vi "Main Menu - Behavioral Study.vi"() -> ()   [LabVIEW 2012]
uses:
  subVIs/Global_var.vi
  <userlib>/dhd_sdk7/dhd_sdk7.lvlib
panel:
  out "Please wait...":u16(slide) scale=0.0..2000.0
  in  "step4":bool
  in  "Setting":bool
  in  "step3":bool
  in  "step2":bool
  out "error out":errorcluster
  out "stripped path":path
  out "DeviceID":bool
  in  "step1":bool
  in  "stop":bool
  out "Patient's ID":string
  # "Somatosensory Training Protocol\n\n(coded by ananda)  ver1.3, April 2017"
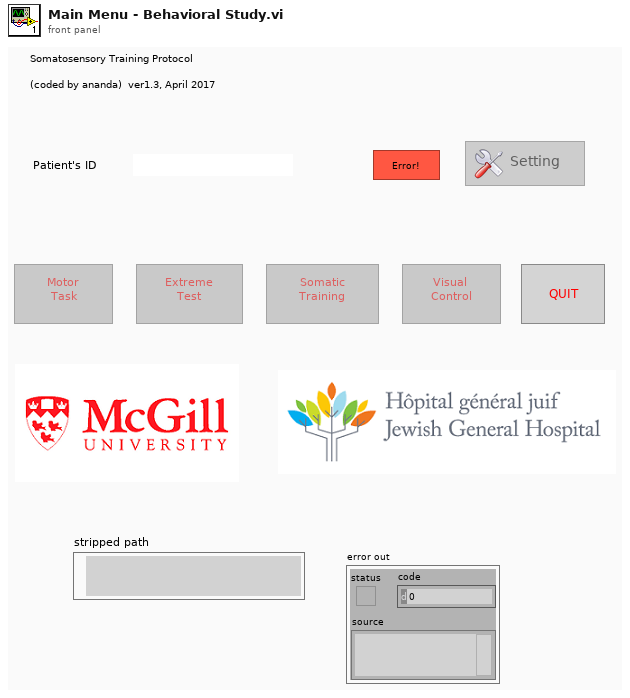
[diagram p1: front panel]
types:
  T1 = enum8{"Enabled", "Disabled", "Disabled and Grayed Out"}
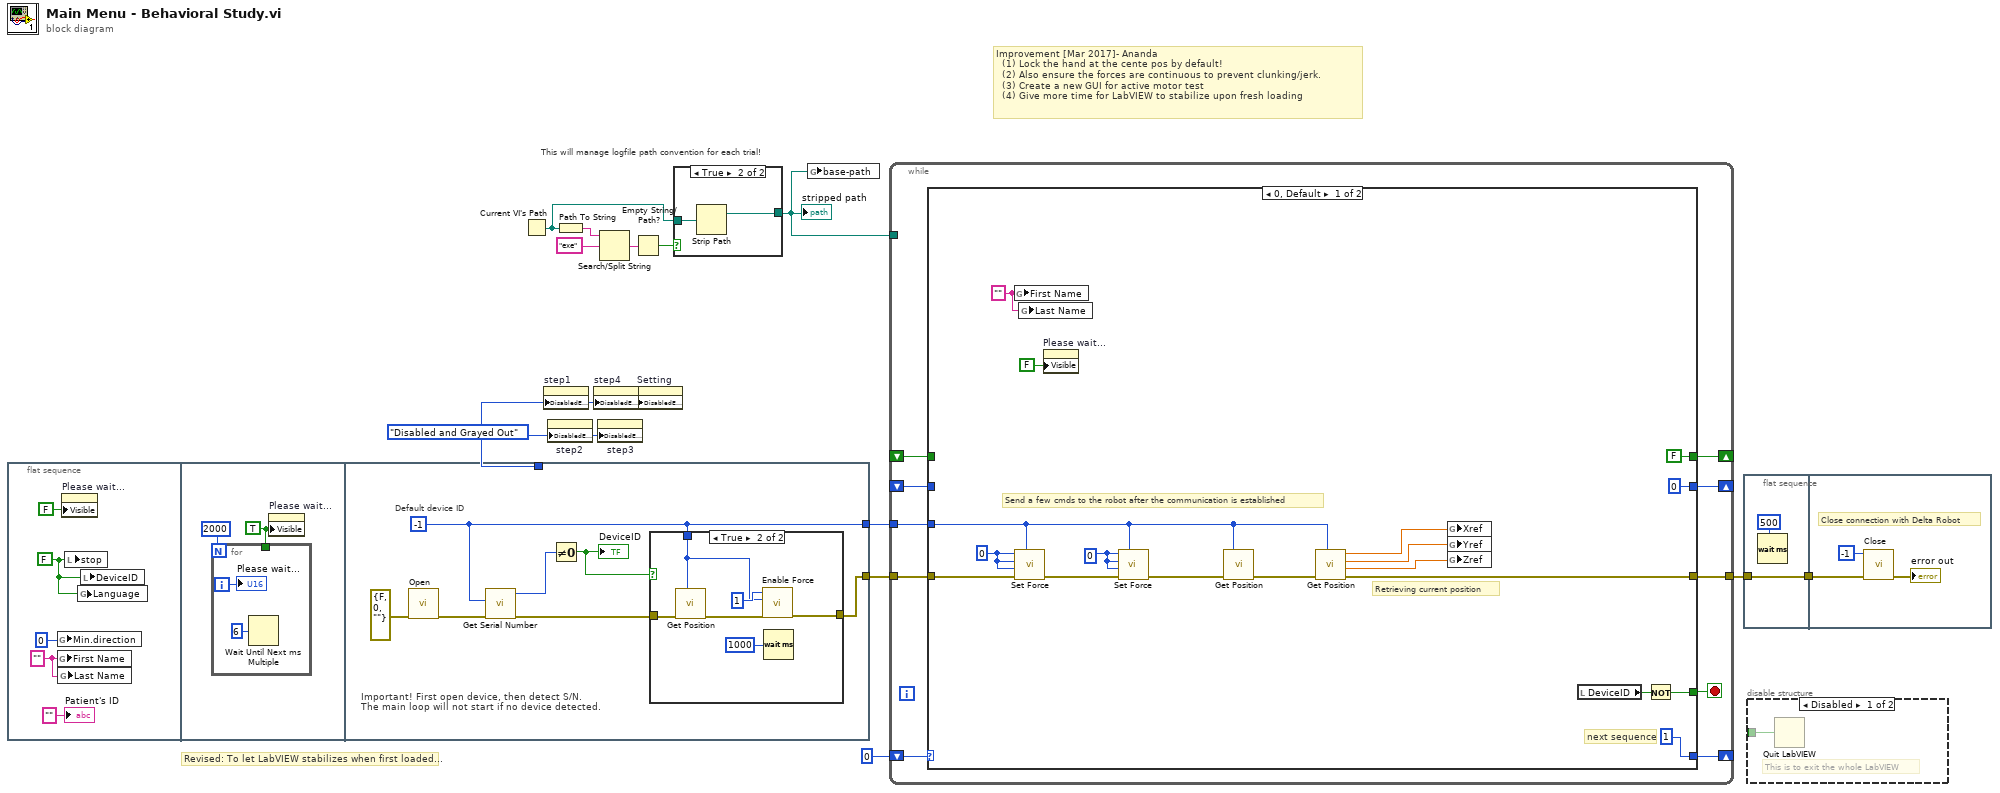
[diagram p0: block diagram]
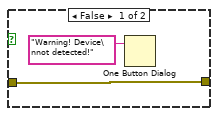
[diagram p2: hidden frame]
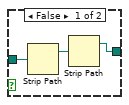
[diagram p4: hidden frame]
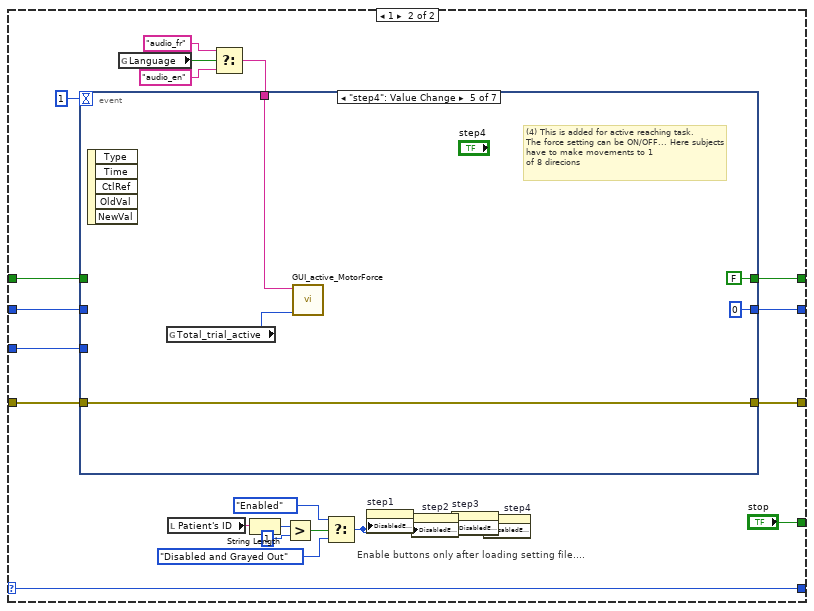
[diagram p5: hidden frame]
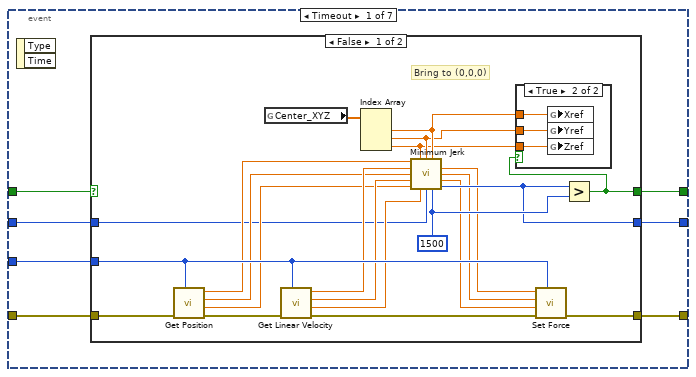
[diagram p6: hidden frame]
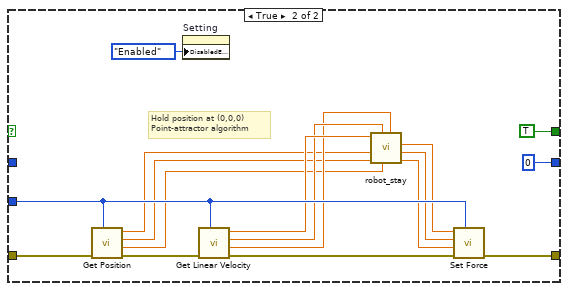
[diagram p8: hidden frame]
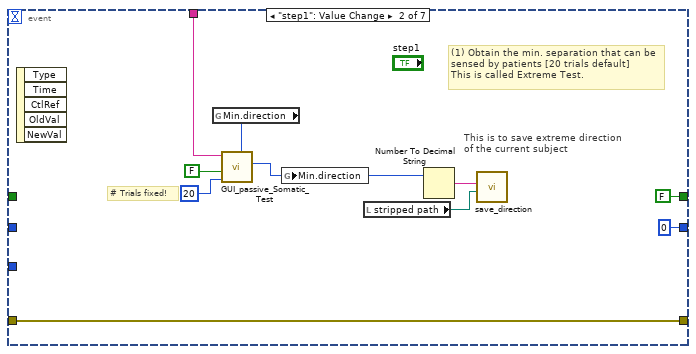
[diagram p9: hidden frame]
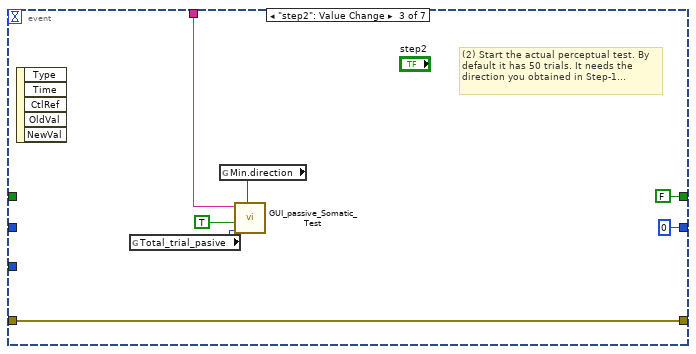
[diagram p10: hidden frame]
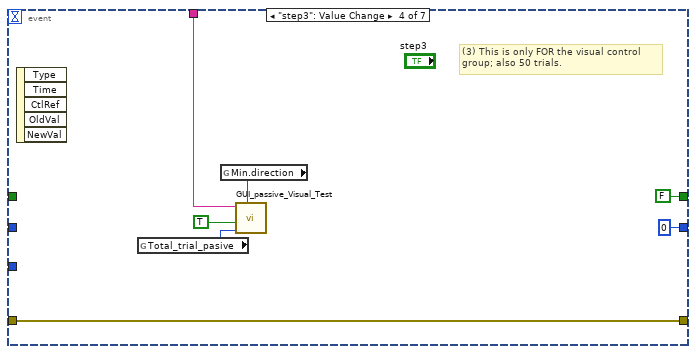
[diagram p11: hidden frame]
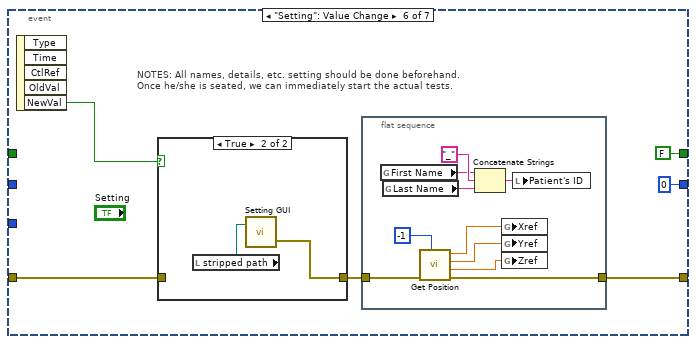
[diagram p12: hidden frame]
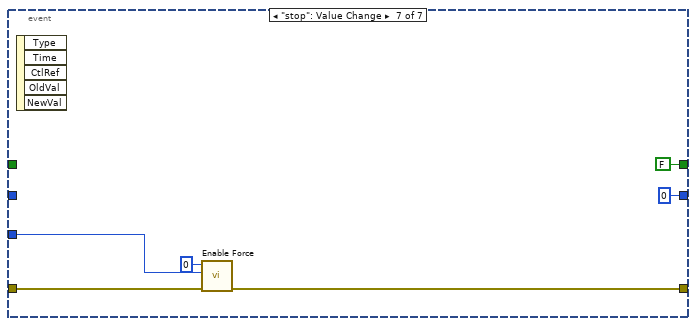
[diagram p14: hidden frame]
diagram:
  w3 = T1."Disabled and Grayed Out" ("Disabled")
  # "Revised: To let LabVIEW stabilizes when first loaded..."
  # "Improvement [Mar 2017]- Ananda\n  (1) Lock the hand at the cente pos by default! \n  (2) Also ensure the forces are continuous to prevent clunking/jerk.\n  (3) Create a new GUI for active motor test\n  (4) Give more time for LabVIEW to stabilize upon fresh loading"
  # "This will manage logfile path convention for each trial!"
  n1 = flat-sequence {
    tunnel: [w22] -> w2
    tunnel: [w23] -> w1
    tunnel: w3 -> [_]
    frame #0 {
      w14 = "" ("Message")
      w16 = FALSE ("stop")
      n2 = global write "Global_var.vi" "Min.direction"(u8 0 ("Extreme Direction")) -> ()
      n3 = global write "Global_var.vi" "First Name"(w14) -> ()
      n4 = global write "Global_var.vi" "Last Name"(w14) -> ()
      n5 = property on="Please wait..." class="Slide (strict)"("Visible"=FALSE) -> ()  [unwired: 2 in, 2 out]
      n6 = local write "stop"(w16) -> ()
      n7 = global write "Global_var.vi" "Language"(w16) -> ()
      n8 = local write "DeviceID"(w16) -> ()
      "Patient's ID" <- "" ("Patient's ID")
    }
    frame #1 {
      w19 = TRUE ("Visible")
      n9 = for {
        N: 2000 -> [_]
        tunnel: w19 -> [_]
        i -> [w20]
        n10 = Wait Until Next ms Multiple(millisecond multiple=u32 6) -> ()  [unwired: 1 out]
        "Please wait..." <- w20
      }
      n11 = property on="Please wait..." class="Slide (strict)"("Visible"=w19) -> ()  [unwired: 2 in, 2 out]
    }
    frame #2 {
      w22 = i8 -1 ("function return")
      # "Important! First open device, then detect S/N. \nThe main loop will not start if no device detected."
      # "Default device ID"
      n12 = call <userlib>:"Open.vi"("error in (no error)"=errorcluster {"status"=FALSE, "code"=0, "source"=""}) -> ("error out"=w27:errorcluster)  [unwired: 9 in, 1 out]
      n13 = call <userlib>:"Get Serial Number.vi"("error in (no error)"=w27, "ID"=w22) -> ("error out"=w24:errorcluster, "sn out"=w26:u16)  [unwired: 7 in, 1 out]
      n14 = Not Equal To 0?(x=w26) -> (x != 0?=w25:bool)
      "DeviceID" <- w25
      n15 = case shown="True" w25 {
        tunnel: w24 -> [w30 w34]
        tunnel: [w30 w33] -> w23
        tunnel: w22 -> [_ w32]
        frame False {
          n16 = One Button Dialog(message="Warning! Device\nnot detected!") -> ()  [unwired: 1 in, 1 out]
        }
        frame True {
          n17 = call <userlib>:"Get Position.vi"("ID"=w32, "error in (no error)"=w34) -> ("error out"=w35:errorcluster)  [unwired: 5 in, 4 out]
          n18 = call <userlib>:"Enable Force.vi"("error in (no error)"=w35, "ID"=w32, "val"=u8 1) -> ("error out"=w33:errorcluster)  [unwired: 7 in, 1 out]
          n19 = Wait (ms)(milliseconds to wait=u32 1000) -> ()  [unwired: 1 out]
        }
      }
    }
  }
  n20 = Current VI's Path() -> (path=w9:path)
  n21 = property on="step1" class="Bool"("DisabledEnum"=w3) -> ()  [unwired: 2 in, 2 out]
  n22 = property on="step2" class="Bool"("DisabledEnum"=w3) -> ()  [unwired: 2 in, 2 out]
  n23 = Path To String(path=w9) -> (string=w10:string)
  n24 = property on="step4" class="Bool"("DisabledEnum"=w3) -> ()  [unwired: 2 in, 2 out]
  n25 = property on="step3" class="Bool"("DisabledEnum"=w3) -> ()  [unwired: 2 in, 2 out]
  n26 = Search/Split String(string=w10, search string/char (-)="exe" ("regular expression")) -> (match + rest of string=w8:string)  [unwired: 1 in, 2 out]
  n27 = Empty String/Path?(string/path=w8) -> (empty?=w12:bool)
  n28 = property on="Setting" class="Bool"("DisabledEnum"=w3) -> ()  [unwired: 2 in, 2 out]
  n29 = case shown="True" w12 {
    tunnel: w9 -> [w39 w41]
    tunnel: [w37 w40] -> w4
    frame False {
      n30 = Strip Path(path=w39) -> (stripped path=w38:path)  [unwired: 1 out]
      n31 = Strip Path(path=w38) -> (stripped path=w37:path)  [unwired: 1 out]
    }
    frame True {
      n32 = Strip Path(path=w41) -> (stripped path=w40:path)  [unwired: 1 out]
    }
  }
  "stripped path" <- w4
  n33 = global write "Global_var.vi" "base-path"(w4) -> ()
  n34 = while {
    shift-right: [w50] -> _
    shift-left: 0 -> [w51]
    tunnel: w4 -> [_]
    tunnel: w2 -> [w48]
    shift-right: [w47] -> _
    shift-left: _ -> [w46]
    shift-right: [w45] -> _
    shift-left: _ -> [w44]
    tunnel: w1 -> [w43]
    tunnel: [w42] -> w5
    stop <- w49 stop-if-true
    n35 = case shown="0, Default" w51 {
      selector: w51 -> [_ w90]
      tunnel: [1 w90] -> w50
      tunnel: [w68 "stop"] -> w49
      tunnel: w43 -> [w58 w83]
      tunnel: w48 -> [w52 w82]
      tunnel: [w66 w81] -> w42
      tunnel: w46 -> [_ w80]
      tunnel: [u16 0 ("n out") w79] -> w47
      tunnel: [FALSE w78] -> w45
      tunnel: w44 -> [_ w77]
      frame 0, Default {
        w55 = u8 0 ("val")
        w59 = "" ("First Name")
        w57 = u8 0 ("val")
        # "Send a few cmds to the robot after the communication is established"
        # "next sequence"
        # "Retrieving current position"
        n36 = global write "Global_var.vi" "First Name"(w59) -> ()
        n37 = call <userlib>:"Set Force.vi"("ID"=w52, "error in (no error)"=w58, "fz"=w57, "fy"=w57, "fx"=w57) -> ("error out"=w56:errorcluster)  [unwired: 5 in, 1 out]
        n38 = global write "Global_var.vi" "Last Name"(w59) -> ()
        n39 = property on="Please wait..." class="Slide (strict)"("Visible"=FALSE) -> ()  [unwired: 2 in, 2 out]
        n40 = call <userlib>:"Set Force.vi"("ID"=w52, "error in (no error)"=w56, "fz"=w55, "fy"=w55, "fx"=w55) -> ("error out"=w54:errorcluster)  [unwired: 5 in, 1 out]
        n41 = call <userlib>:"Get Position.vi"("ID"=w52, "error in (no error)"=w54) -> ("error out"=w53:errorcluster)  [unwired: 5 in, 4 out]
        n42 = call <userlib>:"Get Position.vi"("ID"=w52, "error in (no error)"=w53) -> ("error out"=w66:errorcluster, "pz out"=w61:dbl, "py out"=w62:dbl, "px out"=w63:dbl)  [unwired: 5 in, 1 out]
        n43 = global write "Global_var.vi" "Xref"(w63) -> ()
        n44 = global write "Global_var.vi" "Yref"(w62) -> ()
        n45 = global write "Global_var.vi" "Zref"(w61) -> ()
        n46 = local read "DeviceID"() -> (w65:bool)
        n47 = Not(x=w65) -> (.not. x?=w68:bool)
      }
      frame 1 {
        # "Enable buttons only after loading setting file...."
        n48 = global read "Global_var.vi" "Language"() -> (w85:bool)
        n49 = local read "Patient's ID"() -> (w70:string)
        n50 = Select(t="audio_fr" ("regular expression"), s=w85, f="audio_en" ("regular expression")) -> (s? t:f=w88:string)
        n51 = event shown="[4] \"step4\": Value Change" {
          selector: _ -> [_ _ _ _ _ _ _]
          dyn-events: _ -> [_ _ _ _ _ _ _]
          timeout: 1 -> [_ _ _ _ _ _ _]
          tunnel: w88 -> [_ w147 w154 w161 w166 _ _]
          tunnel: w83 -> [w97 w140 w151 w158 w165 w171 w190]
          tunnel: w82 -> [w96 _ _ _ _ _ w189]
          tunnel: [w95 w140 w151 w158 w165 w169 w191] -> w81
          tunnel: w80 -> [w94 _ _ _ _ _ _]
          tunnel: [w93 u16 0 ("n out") u16 0 ("n out") u16 0 ("n out") u16 0 ("n out") u16 0 ("n out") u16 0 ("n out")] -> w79
          tunnel: [w92 FALSE FALSE FALSE FALSE FALSE FALSE] -> w78
          tunnel: w77 -> [w91 _ _ _ _ _ _]
          event Timeout {
            n52 = event-data() -> ()  [unwired: 1 in, 2 out]
            n53 = case shown="False" w91 {
              tunnel: w97 -> [w118 w138]
              tunnel: w96 -> [w116 w136]
              tunnel: [w115 w135] -> w95
              tunnel: w94 -> [w108 _]
              tunnel: [w106 u16 0 ("n out")] -> w93
              tunnel: [w101 TRUE] -> w92
              frame False {
                w107 = u16 1500 ("duration")
                # "Bring to (0,0,0)"
                n54 = call <userlib>:"Get Position.vi"("ID"=w116, "error in (no error)"=w118) -> ("error out"=w119:errorcluster, "pz out"=w110:dbl, "py out"=w112:dbl, "px out"=w114:dbl)  [unwired: 5 in, 1 out]
                n55 = global read "Global_var.vi" "Center_XYZ"() -> (w102:dbl[])
                n56 = call <userlib>:"Get Linear Velocity.vi"("ID"=w116, "error in (no error)"=w119) -> ("error out"=w117:errorcluster, "vz out"=w109:dbl, "vy out"=w111:dbl, "vx out"=w113:dbl)  [unwired: 5 in, 1 out]
                n57 = Index Array(array=w102) -> (element #1=w100:dbl, element #2=w99:dbl, element #3=w98:dbl)  [unwired: 3 in]
                n58 = call "Minimum Jerk.vi"("X"=w114, "Xfinal"=w98, "Yfinal"=w99, "Zfinal"=w100, "Vx"=w113, "Y"=w112, "Vy"=w111, "Z"=w110, "Vz"=w109, "current_n"=w108, "duration"=w107) -> ("Fx"=w105:dbl, "Fy"=w104:dbl, "Fz"=w103:dbl, "n out"=w106:u16)  [unwired: 1 out]
                n59 = call <userlib>:"Set Force.vi"("ID"=w116, "error in (no error)"=w117, "fz"=w103, "fy"=w104, "fx"=w105) -> ("error out"=w115:errorcluster)  [unwired: 5 in, 1 out]
                n60 = Greater?(x=w106, y=w107) -> (0:w101:bool)
                n61 = case shown="True" w101 {
                  tunnel: w100 -> [_ w122]
                  tunnel: w99 -> [_ w121]
                  tunnel: w98 -> [_ w120]
                  frame False {
                  }
                  frame True {
                    n62 = global write "Global_var.vi" "Xref"(w122) -> ()
                    n63 = global write "Global_var.vi" "Yref"(w121) -> ()
                    n64 = global write "Global_var.vi" "Zref"(w120) -> ()
                  }
                }
              }
              frame True {
                # "Hold position at (0,0,0)\nPoint-attractor algorithm"
                n65 = call <userlib>:"Get Position.vi"("ID"=w136, "error in (no error)"=w138) -> ("error out"=w139:errorcluster, "pz out"=w124:dbl, "py out"=w125:dbl, "px out"=w126:dbl)  [unwired: 5 in, 1 out]
                n66 = property on="Setting" class="Bool"("DisabledEnum"=T1."Enabled" ("Disabled")) -> ()  [unwired: 2 in, 2 out]
                n67 = call <userlib>:"Get Linear Velocity.vi"("ID"=w136, "error in (no error)"=w139) -> ("error out"=w137:errorcluster, "vz out"=w127:dbl, "vy out"=w128:dbl, "vx out"=w129:dbl)  [unwired: 5 in, 1 out]
                n68 = call "robot_stay.vi"("Vz"=w127, "Z"=w124, "Vy"=w128, "Y"=w125, "X"=w126, "Vx"=w129) -> ("Fz"=w131:dbl, "Fy"=w132:dbl, "Fx"=w133:dbl)  [unwired: 3 in]
                n69 = call <userlib>:"Set Force.vi"("ID"=w136, "error in (no error)"=w137, "fz"=w131, "fy"=w132, "fx"=w133) -> ("error out"=w135:errorcluster)  [unwired: 5 in, 1 out]
              }
            }
          }
          event "step1": Value Change {
            # "This is to save extreme direction of the current subject"
            # "# Trials fixed!"
            # "(1) Obtain the min. separation that can be sensed by patients [20 trials default]\nThis is called Extreme Test."
            n70 = event-data() -> ()  [unwired: 1 in, 5 out]
            n71 = global read "Global_var.vi" "Min.direction"() -> (w142:i8)
            n72 = call "GUI_passive_Somatic_Test.vi"("lang"=w147, "Do test?"=FALSE, "Total trial"=u16 20, "Direction"=w142) -> ("Direction 2"=w144:i8)  [unwired: 4 in, 1 out]
            n73 = global write "Global_var.vi" "Min.direction"(w144) -> ()
            n74 = local read "stripped path"() -> (w143:path)
            n75 = Number To Decimal String(number=w144) -> (decimal integer string=w141:string)  [unwired: 1 in]
            n76 = call "save_direction.vi"("Path"=w143, "Direction"=w141) -> ()  [unwired: 10 in]
          }
          event "step2": Value Change {
            # "(2) Start the actual perceptual test. By default it has 50 trials. It needs the direction you obtained in Step-1..."
            n77 = event-data() -> ()  [unwired: 1 in, 5 out]
            n78 = global read "Global_var.vi" "Total_trial_pasive"() -> (w152:u8)
            n79 = global read "Global_var.vi" "Min.direction"() -> (w150:i8)
            n80 = call "GUI_passive_Somatic_Test.vi"("lang"=w154, "Do test?"=TRUE, "Total trial"=w152, "Direction"=w150) -> ()  [unwired: 4 in, 2 out]
          }
          event "step3": Value Change {
            # "(3) This is only FOR the visual control group; also 50 trials."
            n81 = event-data() -> ()  [unwired: 1 in, 5 out]
            n82 = global read "Global_var.vi" "Total_trial_pasive"() -> (w159:u8)
            n83 = global read "Global_var.vi" "Min.direction"() -> (w157:i8)
            n84 = call "GUI_passive_Visual_Test.vi"("Direction"=w157, "Total trial"=w159, "Do test?"=TRUE, "lang"=w161) -> ()  [unwired: 7 in, 1 out]
          }
          event "step4": Value Change {
            # "(4) This is added for active reaching task.\nThe force setting can be ON/OFF... Here subjects have to make movements to 1\nof 8 direcions"
            n85 = event-data() -> ()  [unwired: 1 in, 5 out]
            n86 = global read "Global_var.vi" "Total_trial_active"() -> (w164:u8)
            n87 = call "GUI_active_MotorForce.vi"("lang"=w166, "Total trial"=w164) -> ()  [unwired: 7 in, 1 out]
          }
          event "Setting": Value Change {
            # "NOTES: All names, details, etc. setting should be done beforehand.\nOnce he/she is seated, we can immediately start the actual tests."
            n88 = event-data() -> ("NewVal"=w172:bool)  [unwired: 1 in, 4 out]
            n89 = case shown="True" w172 {
              tunnel: [w185 w186] -> w170
              tunnel: w171 -> [w185 _]
              frame False {
              }
              frame True {
                n90 = local read "stripped path"() -> (w187:path)
                n91 = call "Setting GUI.vi"("Path_In"=w187) -> ("error out"=w186:errorcluster)  [unwired: 2 in]
              }
            }
            n92 = flat-sequence {
              tunnel: w170 -> [w184]
              tunnel: [w183] -> w169
              frame #0 {
                n93 = global read "Global_var.vi" "First Name"() -> (w176:string)
                n94 = global read "Global_var.vi" "Last Name"() -> (w178:string)
                n95 = call <userlib>:"Get Position.vi"("ID"=i8 -1, "error in (no error)"=w184) -> ("error out"=w183:errorcluster, "pz out"=w179:dbl, "py out"=w181:dbl, "px out"=w182:dbl)  [unwired: 5 in, 1 out]
                n96 = Concatenate Strings(w176, "_" ("string"), w178) -> (w175:string)
                n97 = global write "Global_var.vi" "Xref"(w182) -> ()
                n98 = global write "Global_var.vi" "Yref"(w181) -> ()
                n99 = global write "Global_var.vi" "Zref"(w179) -> ()
                n100 = local write "Patient's ID"(w175) -> ()
              }
            }
          }
          event "stop": Value Change {
            n101 = event-data() -> ()  [unwired: 1 in, 5 out]
            n102 = call <userlib>:"Enable Force.vi"("error in (no error)"=w190, "ID"=w189, "val"=u8 0) -> ("error out"=w191:errorcluster)  [unwired: 7 in, 1 out]
          }
        }
        n103 = String Length(string=w70) -> (length=w71:i32)
        n104 = Greater?(x=w71, y=1) -> (0:w73:bool)
        n105 = Select(t=T1."Enabled" ("Disabled"), s=w73, f=T1."Disabled and Grayed Out" ("Disabled")) -> (s? t:f=w76:T1)
        n106 = property on="step1" class="Bool"("DisabledEnum"=w76) -> ()  [unwired: 2 in, 2 out]
        n107 = property on="step2" class="Bool"("DisabledEnum"=w76) -> ()  [unwired: 2 in, 2 out]
        n108 = property on="step3" class="Bool"("DisabledEnum"=w76) -> ()  [unwired: 2 in, 2 out]
        n109 = property on="step4" class="Bool"("DisabledEnum"=w76) -> ()  [unwired: 2 in, 2 out]
      }
    }
  }
  n110 = flat-sequence {
    tunnel: w5 -> [w194]
    tunnel: [w194] -> w7
    tunnel: w7 -> [w196]
    frame #0 {
      n111 = Wait (ms)(milliseconds to wait=u32 500) -> ()  [unwired: 1 out]
    }
    frame #1 {
      # "Close connection with Delta Robot"
      n112 = call <userlib>:"Close.vi"("error in (no error)"=w196, "ID"=i8 -1) -> ("error out"=→"error out":errorcluster)  [unwired: 8 in, 1 out]
    }
  }
  n113 = disable-structure shown="Disabled" {
    disable-tunnel: _ -> [w199 _]
    frame Disabled {
      # "This is to exit the whole LabVIEW"
      n114 = Quit LabVIEW(quit? (T)=w199) -> ()
    }
    frame Enabled {
    }
  }
